vi "Initialize.vi"(8 "error in (no error)":errorcluster, 11 "Fault Monitor in":refnum<class "Fault Monitor.lvclass">) -> (0 "error out":errorcluster, 3 "Fault Monitor out":refnum<class "Fault Monitor.lvclass">)   [LabVIEW 2023, in "Fault Monitor.lvlib" / "Fault Monitor.lvclass"]
doc: "<b>Initialize</b>\nThis routine is implemented in the Pre-Launch Init override -> as a result, it is not necessary to call initialize anywhere else, and any methods that need to be called after post-launch intiialize can be implemented here.\n\n<b>Engine</b> - Calls Check for Errors"
uses:
  Library/Fault Monitor.lvclass
  builds/Main/Docking.lvlibp/Bottom Panel/BottomDock.lvclass
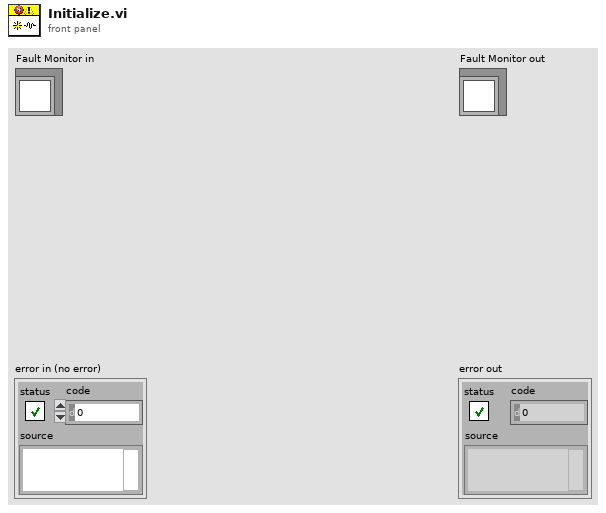
[diagram p1: front panel]
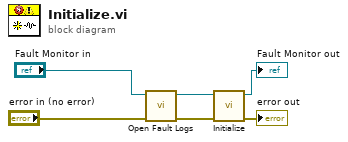
[diagram p0: block diagram]
diagram:
  n1 = call "Open Fault Logs.vi"("error in (no error)"="error in (no error)", "Fault Monitor in"="Fault Monitor in") -> ("error out"=w2:errorcluster, "Fault Monitor out"=w1:refnum<class "Fault Monitor.lvclass">)  [unwired: 8 in]
  n2 = call-parent "Initialize.vi"("error in (no error)"=w2, "Engine in"=w1) -> ("error out"=→"error out":errorcluster, "Engine out"=→"Fault Monitor out":refnum<class "Fault Monitor.lvclass">)  [unwired: 8 in]
